vi "S2C_XML_CreateMeasMeta.vi"(8 "Error In":errorcluster, 11 "MetaArray":cluster{"MetaName":string, "MetaValue":string}[](array[cluster])) -> (0 "Error Out":errorcluster)   [LabVIEW 2015]
uses:
  S2C_XML_Globals.vi
  <vilib>/xml/Close Reference(Node).vi
  <resource>/objmgr/DOMUserDefRef.rc
  <vilib>/xml/NI_XML.lvlib
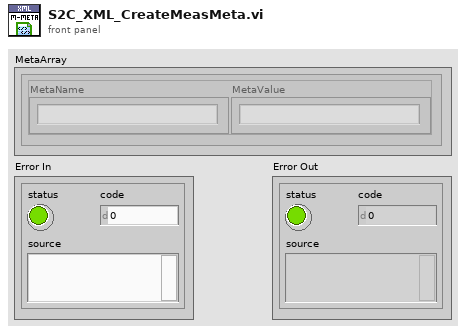
[diagram p1: front panel]
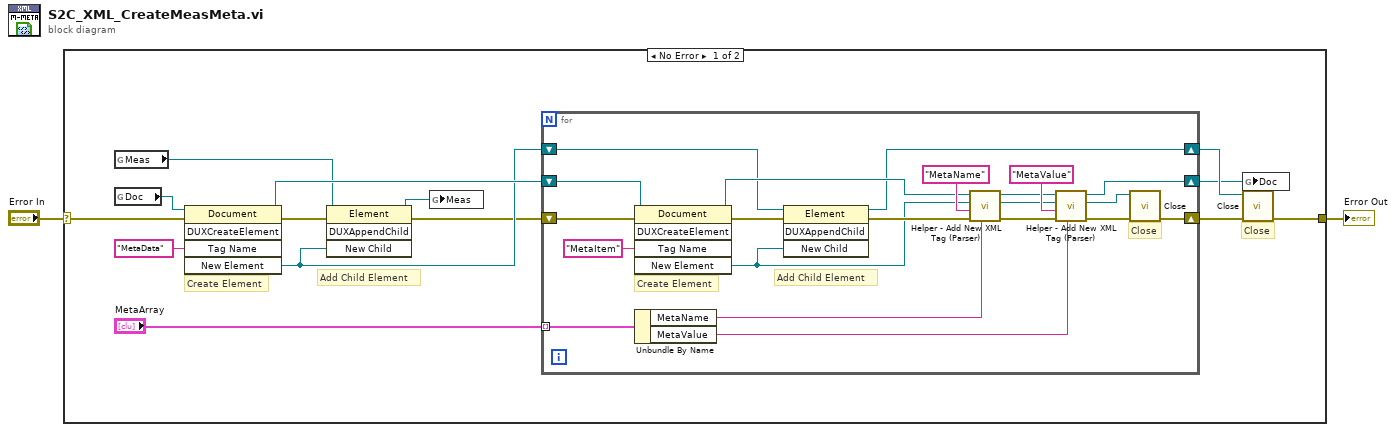
[diagram p0: block diagram]
diagram:
  n1 = case shown="No Error" "Error In" {
    selector: "Error In" -> [w15 w38]
    tunnel: [w11 w38] -> w2
    frame No Error {
      # "Close"
      # "Add Child Element"
      # "Create Element"
      n2 = global read "S2C_XML_Globals.vi" "Meas"() -> (w5:refnum<k20>)
      n3 = global read "S2C_XML_Globals.vi" "Doc"() -> (w6:refnum<k20>)
      n4 = invoke class="Document" method="DUXCreateElement"(reference=w6, error in=w15, "Tag Name"="MetaData") -> (reference out=w14:refnum<k20>, error out=w13:errorcluster, "New Element"=w10:refnum<k20>)  [unwired: 2 in, 2 out]
      n5 = invoke class="Element" method="DUXAppendChild"(reference=w5, error in=w13, "New Child"=w10) -> (reference out=w4:refnum<k20>, error out=w7:errorcluster)  [unwired: 1 in, 2 out]
      n6 = global write "S2C_XML_Globals.vi" "Meas"(w4) -> ()
      n7 = for {
        tunnel: "MetaArray" -> [w37] mode=indexing
        shift-right: [w26] -> w3
        shift-left: w14 -> [w29]
        shift-right: [w21] -> w9
        shift-left: w10 -> [w25]
        shift-right: [w17] -> w8
        shift-left: w7 -> [w24]
        # "Add Child Element"
        # "Close"
        # "Create Element"
        n8 = invoke class="Document" method="DUXCreateElement"(reference=w29, error in=w24, "Tag Name"="MetaItem") -> (reference out=w27:refnum<k20>, error out=w20:errorcluster, "New Element"=w22:refnum<k20>)  [unwired: 2 in, 2 out]
        n9 = Unbundle By Name(w37) -> ("MetaName"=w35:string, "MetaValue"=w30:string)
        n10 = invoke class="Element" method="DUXAppendChild"(reference=w25, error in=w20, "New Child"=w22) -> (reference out=w21:refnum<k20>, error out=w23:errorcluster)  [unwired: 1 in, 2 out]
        n11 = call "Helper - Add New XML Tag (Parser).vi"("Tag Data"=w35, "error in (no error)"=w23, "Tag Name"="MetaName", "Owning Element"=w22, "DOM document"=w27) -> ("error out"=w31:errorcluster, "dup Owning Element"=w32:refnum<k20>, "dup DOM document"=w33:refnum<k20>)  [unwired: 4 in]
        n12 = call "Helper - Add New XML Tag (Parser).vi"("Tag Data"=w30, "error in (no error)"=w31, "Tag Name"="MetaValue", "Owning Element"=w32, "DOM document"=w33) -> ("error out"=w19:errorcluster, "dup Owning Element"=w18:refnum<k20>, "dup DOM document"=w26:refnum<k20>)  [unwired: 4 in]
        n13 = call-poly <vilib>:"Close.vi"("error in (no error)"=w19, "node"=w18) -> ("error out"=w17:errorcluster)  [unwired: 7 in]
      }
      n14 = global write "S2C_XML_Globals.vi" "Doc"(w3) -> ()
      n15 = call-poly <vilib>:"Close.vi"("error in (no error)"=w8, "node"=w9) -> ("error out"=w11:errorcluster)  [unwired: 7 in]
    }
    frame Error {
    }
  }
  "Error Out" <- w2
